vi "Count Vision Events.vi"(8 "Event":bool) -> (0 "Count":i32)   [LabVIEW 2015]
uses:
  TypeDefs Dani/Exit FGV Enum Dani.ctl
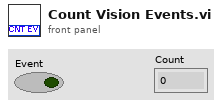
[diagram p1: front panel]
types:
  T1 = typedef "Exit FGV Enum Dani.ctl" = enum16{"Get Count", "Set Count"}
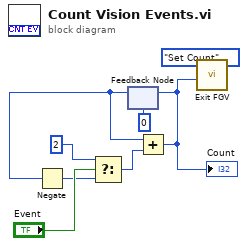
[diagram p0: block diagram]
diagram:
  n1 = feedback #1(0) -> (w3:i32)
  n2 = Negate(x=w3) -> (-x=w1:i32)
  n3 = Select(t=2 ("f"), s="Event", f=w1) -> (s? t:f=w5:i32)
  n4 = Add(x=w3, y=w5) -> (x+y=w7:i32)
  "Count" <- w7
  n5 = feedback-in #1(w7) -> ()
  n6 = call "Exit FGV.vi"("Exit FGV Command"=Exit_FGV_Enum_Dani."Set Count", 9:w7) -> ()  [unwired: 9 in, 1 out]
